vi "Polling Core.vi"(8 "Error In":errorcluster, 11 "CS++SimMotor in":refnum<class "CS++SimMotor.lvclass">) -> (0 "Error Out":errorcluster, 3 "CS++SimMotor out":refnum<class "CS++SimMotor.lvclass">)   [LabVIEW 2015, in "CS++SimMotor.lvlib" / "CS++SimMotor.lvclass"]
uses:
  CS++SimMotor.lvclass
  CSPP_Core/Actors/CS++BaseActor/CS++BaseActor.lvclass/CS++BaseActor.ctl
  CSPP_Core/Actors/CS++BaseActor/CS++BaseActor.lvclass
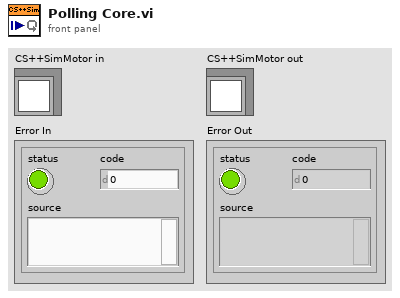
[diagram p1: front panel]
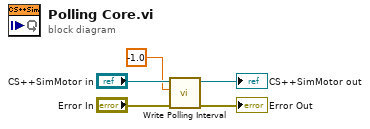
[diagram p0: block diagram]
diagram:
  n1 = call "Write Polling Interval.vi"("error in (no error)"="Error In", "Polling Interval"=dbl[unit] -1.0, "CS++BaseActor in"="CS++SimMotor in") -> ("error out"=→"Error Out":errorcluster, "CS++BaseActor out"=→"CS++SimMotor out":refnum<class "CS++SimMotor.lvclass">)  [unwired: 7 in]
